vi "16 BIT RAM - 1 register.vi"(2 "Hold":bool, 3 "Address":bool[](array[boolean]), 4 "Address of this register":bool[](array[boolean]), 5 "Data In":bool[](array[boolean])=[FALSE, FALSE, FALSE, FALSE, FALSE, FALSE, FALSE, FALSE, FALSE, FALSE, FALSE, FALSE, FALSE, FALSE, FALSE, FALSE], 6 "Clock":bool) -> (0 "z":bool[](array[boolean]))   [LabVIEW 2012]
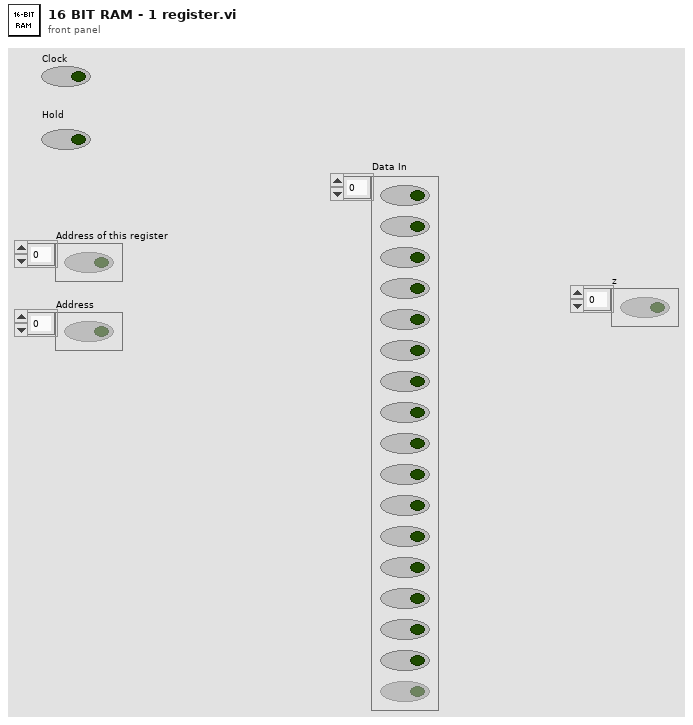
[diagram p1: front panel]
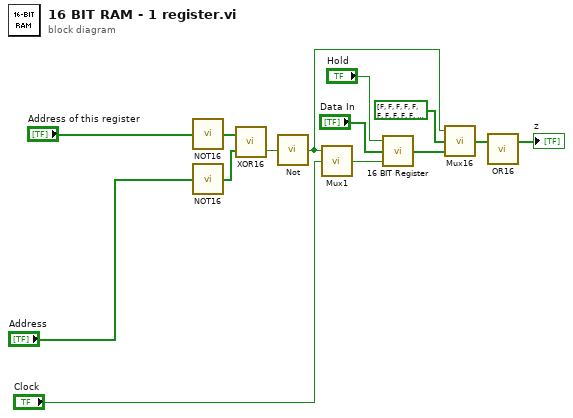
[diagram p0: block diagram]
diagram:
  n1 = call "NOT16.vi"("A"="Address of this register") -> ("z"=w5:bool[])
  n2 = call "NOT16.vi"("A"="Address") -> ("z"=w6:bool[])
  n3 = call "XOR16.vi"("B"=w6, "A"=w5) -> ("compound"=w7:bool)  [unwired: 1 out]
  n4 = call "Not.vi"("In"=w7) -> ("Out"=w8:bool)
  n5 = call "Mux1.vi"("A"="Clock", "s0"=w8) -> ("z"=w3:bool)  [unwired: 1 in]
  n6 = call "16 BIT Register.vi"("Clock"=w3, "Data In"="Data In", "Hold"="Hold") -> ("Data Out"=w12:bool[])
  n7 = call "Mux16.vi"("B"=w12, "A"=bool[] [FALSE, FALSE, FALSE, FALSE, FALSE, FALSE, FALSE, FALSE, FALSE, FALSE, FALSE, FALSE, FALSE, FALSE, FALSE, FALSE] ("B"), "s0"=w8) -> ("z"=w9:bool[])
  n8 = call "OR16.vi"("A"=w9) -> ("z"=→"z":bool[])  [unwired: 1 in, 1 out]
